vi "Greeter SayHello.vi"(6 "contextId":T1, 7 "Occurrence":enum16{"With Occurrence", "Without Occurrence"}(ring), 8 "error in":errorcluster, 9 "timeout (ms)":i32=-1, 10 "Request Data":T3, 11 "gRPC ID":T1) -> (0 "error out":errorcluster, 2 "Response Data":T2, 3 "gRPC ID out":T1)   [LabVIEW 2019, in "helloworld_client.lvlib"]
uses:
  helloworld_client.lvlib
  <vilib>/gRPC/LabVIEW gRPC Library/Shared/grpcId.ctl
  RPC Messages/helloworld_HelloRequest.ctl
  RPC Messages/helloworld_HelloReply.ctl
  RPC Messages/helloworld_HelloReply_Flat.ctl
  14035477-4c25-4107-8ed5-d0c4ef420ce5.vi
  <vilib>/gRPC/LabVIEW gRPC Library/Shared/TranslateGrpcError.vi
  <vilib>/gRPC/LabVIEW gRPC Library/Shared/Wait On Occurence.vi
  <vilib>/gRPC/LabVIEW gRPC Library/Server API/Server/Get Server DLL Path.vi
  <vilib>/Utility/error.llb/Error Cluster From Error Code.vi
  <vilib>/gRPC/LabVIEW gRPC Library/grpc-lvsupport-release.lvlib
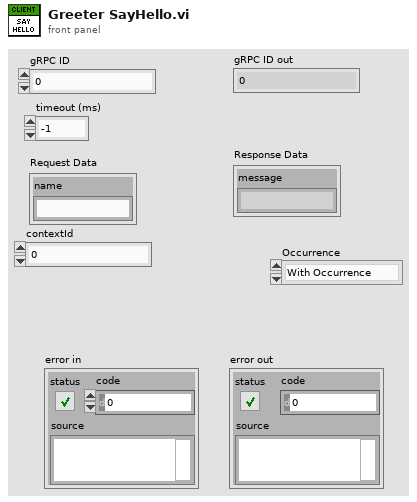
[diagram p1: front panel]
types:
  T1 = typedef "grpc-lvsupport-release.lvlib/grpcId.ctl" = u64
  T2 = typedef "helloworld_client.lvlib/helloworld_HelloReply.ctl" = cluster{"message":string}
  T3 = typedef "helloworld_client.lvlib/helloworld_HelloRequest.ctl" = cluster{"name":string}
  T4 = typedef "helloworld_client.lvlib/helloworld_HelloReply_Flat.ctl" = cluster{"message":string}
  T5 = typedef "helloworld_client.lvlib/helloworld_HelloRequest_Flat.ctl" = cluster{"name":string}
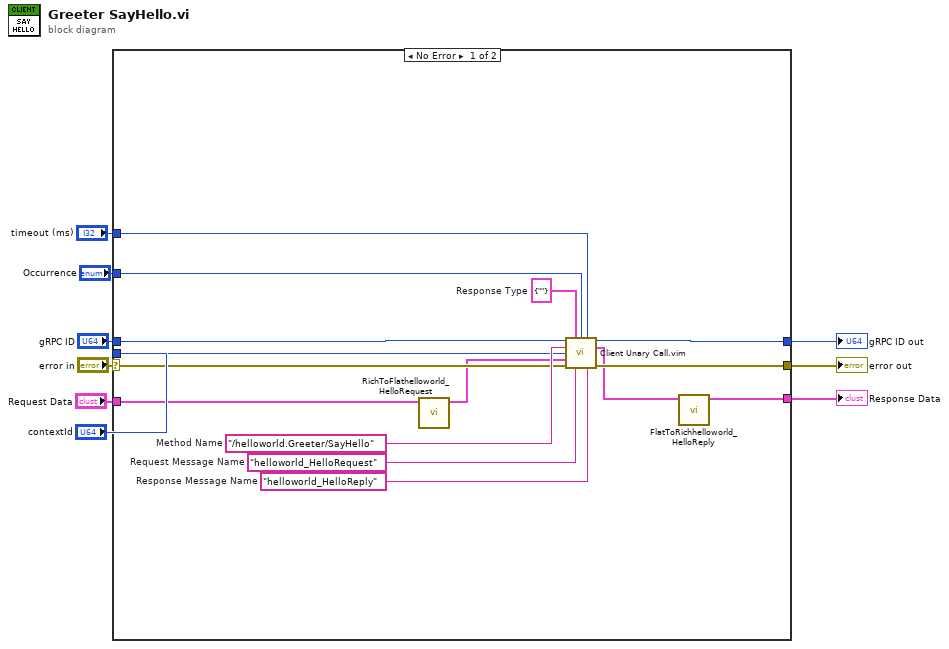
[diagram p0: block diagram]
diagram:
  n1 = case shown="No Error" "error in" {
    selector: "error in" -> [w20 w25]
    tunnel: [w19 w25] -> w8
    tunnel: "gRPC ID" -> [w18 w26]
    tunnel: [w17 w26] -> w6
    tunnel: "Request Data" -> [w14 _]
    tunnel: [w11 _] -> w4
    tunnel: "timeout (ms)" -> [w16 _]
    tunnel: "contextId" -> [w15 _]
    tunnel: "Occurrence" -> [w10 _]
    frame No Error {
      w21 = "helloworld_HelloReply"  # Response Message Name
      w22 = "helloworld_HelloRequest"  # Request Message Name
      w23 = T4 {"message"=""}  # Response Type
      w24 = "/helloworld.Greeter/SayHello"  # Method Name
      n2 = call "RichToFlathelloworld_HelloRequest.vi"("InputCluster"=w14) -> ("OutputCluster"=w13:T5)  [unwired: 10 in]
      n3 = call "Client Unary Call.vim"("ClientID in"=w18, "Response Type"=w23, "Occurrence"=w10, "timeout (ms)"=w16, "Method Name"=w24, "contextId"=w15, "Request Data"=w13, "error in"=w20, "Request Message Name"=w22, "Response Message Name"=w21) -> ("ClientID out"=w17:u64, "Response Data"=w12:T4, "error out"=w19:errorcluster)  [unwired: 3 in]
      n4 = call "FlatToRichhelloworld_HelloReply.vi"("InputCluster"=w12) -> ("OutputCluster"=w11:T2)  [unwired: 10 in]
    }
    frame Error {
    }
  }
  "error out" <- w8
  "gRPC ID out" <- w6
  "Response Data" <- w4
